vi "SRV_PM_Data Byte Unstuffing_02.vi"(0 "Stuffed Data":u8[](array[numeric]) format="%.0x", 1 "Data Length":u32, 11 "error in (no error)":errorcluster) -> (4 "Stuffed Data dup":u8[](array[numeric]) format="%.0x", 8 "Data":u8[](array[numeric]) format="%.0x", 10 "All Data Received?":bool, 14 "Remaining Stuffed Data":u8[](array[numeric]) format="%.0x", 15 "error out":errorcluster)   [LabVIEW 2009]
panel:
  in  "Stuffing Byte (0x00)":u8 format="%.0x"
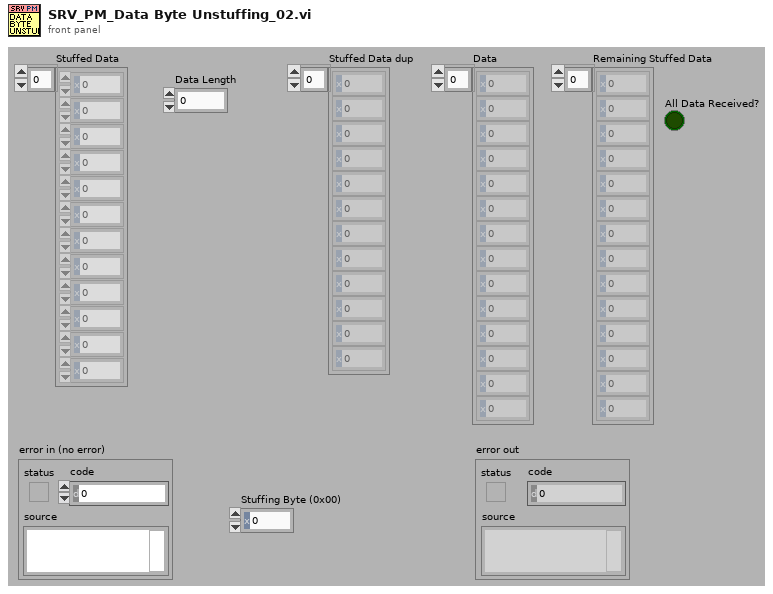
[diagram p1: front panel]
types:
  T1 = typedef "SRV_PM_Packet.ctl" = cluster{"Packet Data":u8[], "Complete?":bool, "Error?":bool}
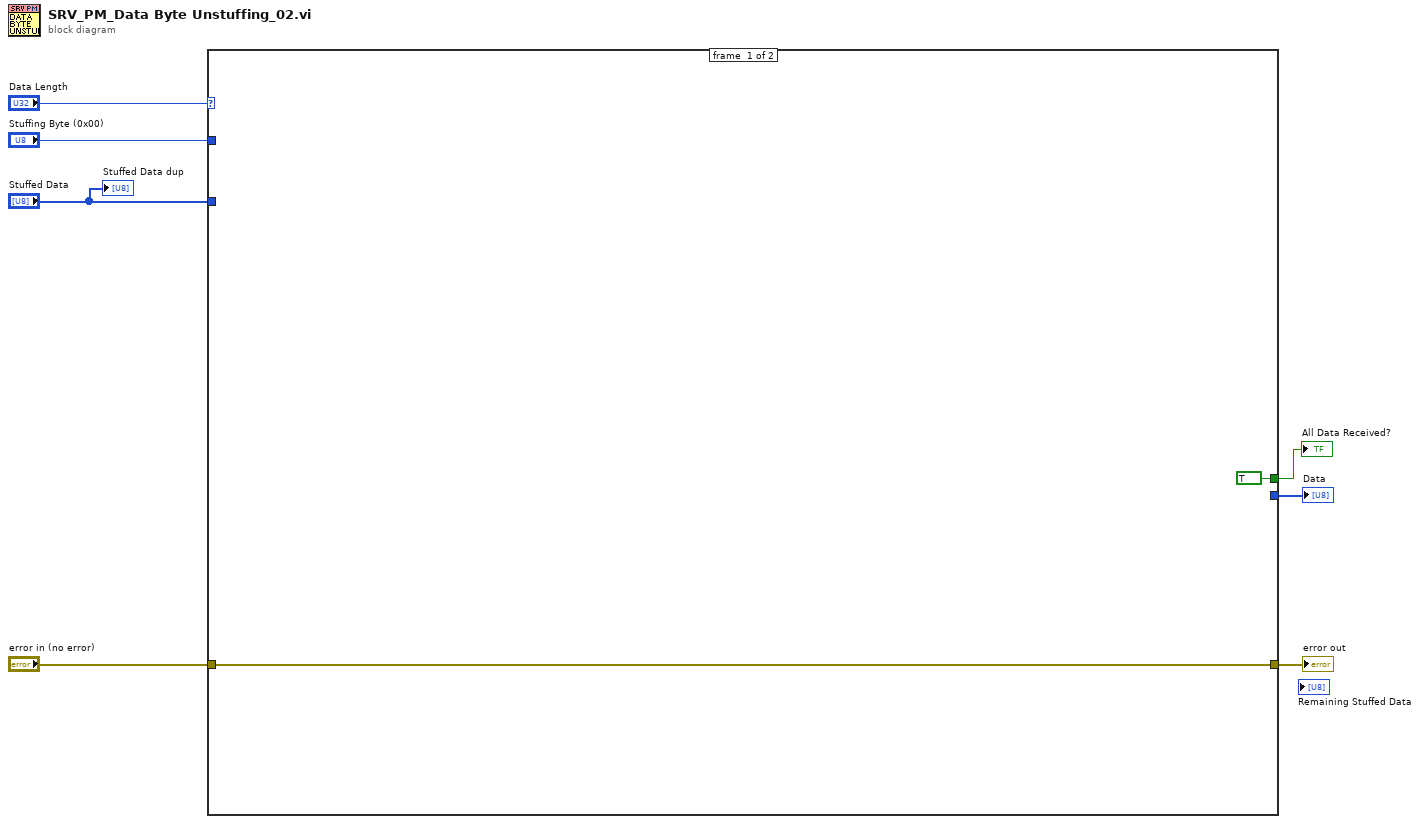
[diagram p0: block diagram]
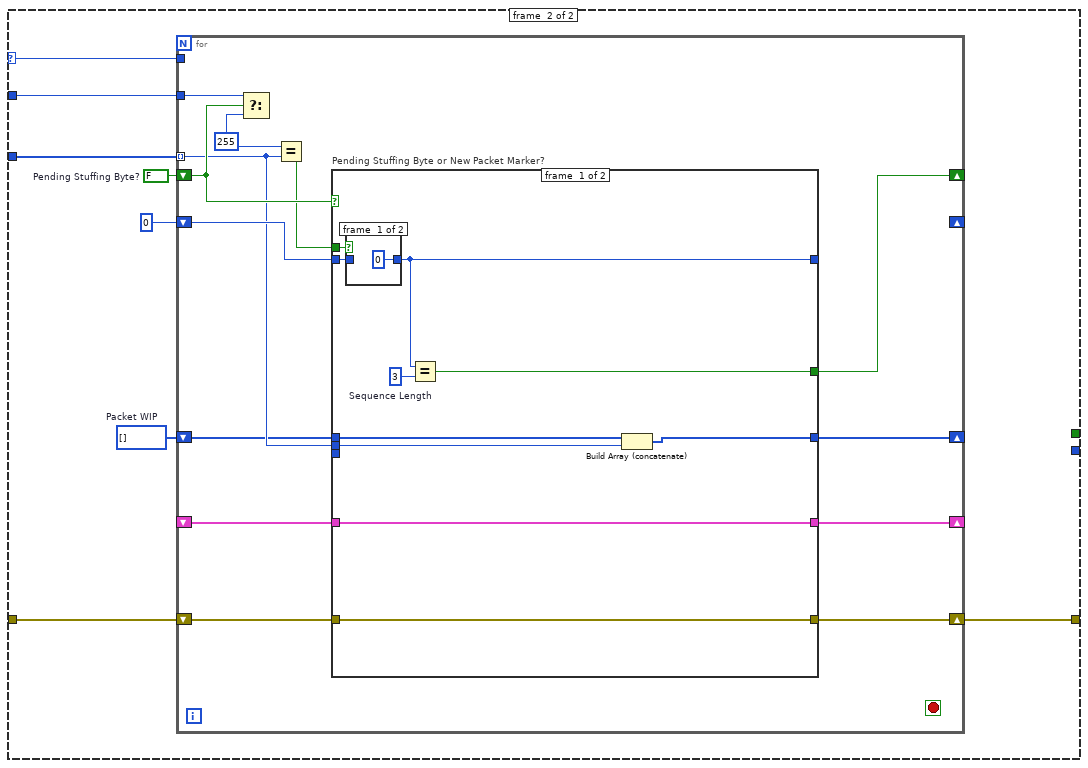
[diagram p2: hidden frame]
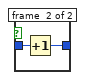
[diagram p3: hidden frame]
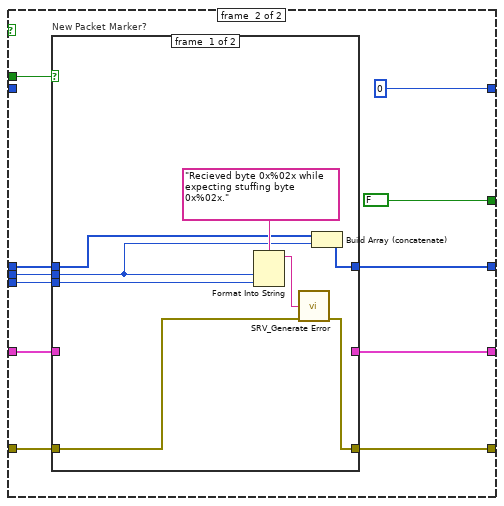
[diagram p4: hidden frame]
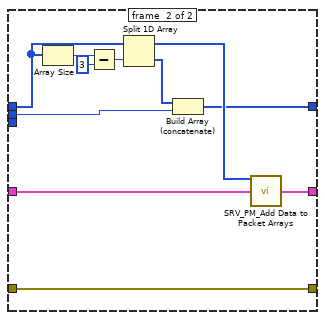
[diagram p5: hidden frame]
diagram:
  n1 = case shown="Default" "Data Length" {
    selector: "Data Length" -> [_ w14]
    tunnel: [_ _] -> w7
    tunnel: "Stuffing Byte (0x00)" -> [_ w17]
    tunnel: "error in (no error)" -> [w9 w16]
    tunnel: [w9 w15] -> w4
    tunnel: "Stuffed Data" -> [w10 w11]
    tunnel: [TRUE _] -> w1
    frame #0 {
    }
    frame #1 {
      w12 = u8[] []  # Packet WIP
      w18 = FALSE  # Pending Stuffing Byte?
      n2 = for {
        shift-right: [w23] -> _
        shift-left: w18 -> [w30]
        tunnel: w17 -> [w31]
        shift-right: [w24] -> w15
        shift-left: w16 -> [w25]
        tunnel: w14 -> [_]
        shift-right: _ -> [_]
        shift-left: 0 -> [w29]
        shift-right: [w19] -> _
        shift-left: w12 -> [w26]
        tunnel: w11 -> [w27] mode=indexing
        shift-right: [w20] -> _
        shift-left: _ -> [w21]
        stop <- _ stop-if-true
        w22 = u8 255
        n3 = Select(t=w31, s=w30, f=w22) -> ()  [unwired: 1 out]
        n4 = Equal?(x=w22, y=w27) -> (x = y?=w28:bool)
        n5 = case "Pending Stuffing Byte or New Packet Marker?" shown="True" w30 {
          tunnel: w28 -> [w41 w55]
          tunnel: w29 -> [w40 _]
          tunnel: [w33 0] -> _
          tunnel: w26 -> [w38 w54]
          tunnel: [w37 w53] -> w19
          tunnel: w27 -> [w36 w48]
          tunnel: [w35 FALSE] -> w23
          tunnel: w25 -> [w34 w50]
          tunnel: [w34 w49] -> w24
          tunnel: _ -> [_ w47]
          tunnel: w21 -> [w32 w46]
          tunnel: [w32 w45] -> w20
          frame #0 {
            w39 = 3  # Sequence Length
            n6 = case shown="True" w41 {
              tunnel: w40 -> [_ w44]
              tunnel: [0 w43] -> w33
              frame #0 {
              }
              frame #1 {
                n7 = Increment(x=w44) -> (x+1=w43:i32)
              }
            }
            n8 = Equal?(x=w33, y=w39) -> (x = y?=w35:bool)
            n9 = Build Array (concatenate)(w38, w36) -> (w37:u8[])
          }
          frame #1 {
            n10 = case "New Packet Marker?" shown="True" w55 {
              tunnel: w54 -> [w57 w70]
              tunnel: [w58 w64] -> w53
              tunnel: w50 -> [w63 w74]
              tunnel: [w62 w74] -> w49
              tunnel: w48 -> [w56 w66]
              tunnel: w47 -> [w60 _]
              tunnel: w46 -> [_ w68]
              tunnel: [_ w67] -> w45
              frame #0 {
                n11 = Format Into String(format string="Recieved byte 0x%02x while expecting stuffing byte 0x%02x.", w56, w60) -> (resulting string=w61:string)  [unwired: 2 in, 1 out]
                n12 = call "SRV_Generate Error.vi"("Message"=w61, "error in (no error)"=w63) -> ("error out"=w62:errorcluster)  [unwired: 13 in]
                n13 = Build Array (concatenate)(w57, w56) -> (w58:u8[])
              }
              frame #1 {
                n14 = Array Size(array=w70) -> (size(s)=w73:i32)
                n15 = Subtract(x=w73, y=3) -> (x-y=w71:i32)
                n16 = Split 1D Array(array=w70, index=w71) -> (first subarray=w69:u8[], second subarray=w65:u8[])
                n17 = Build Array (concatenate)(w65, w66) -> (w64:u8[])
                n18 = call "SRV_PM_Add Data to Packet Arrays.vi"("Previous Packet Data"=w69, "Array of Packets"=w68) -> ("Array of Packets out"=w67:T1[])  [unwired: 13 in]
              }
            }
          }
        }
      }
    }
  }
  "error out" <- w4
  "Data" <- w7
  "All Data Received?" <- w1
  "Stuffed Data dup" <- "Stuffed Data"
